vi "Stop.vi"(8 "error out":errorcluster, 10 "Wait (200ms)":u32=200, 11 "Generic Plugin in":refnum<class "Generic Plugin.lvclass">) -> (0 "error IO":errorcluster, 2 "Stopped Successfully (T) Aborted (F)":bool, 3 "Generic Plugin out":refnum<class "Generic Plugin.lvclass">)   [LabVIEW 2011, in "Generic Plugin.lvclass"]
uses:
  Plugin Template/Generic Plugin.lvclass
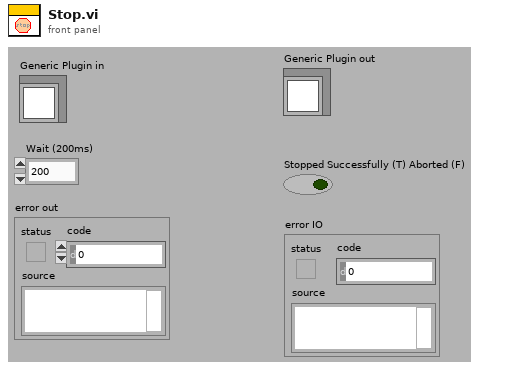
[diagram p1: front panel]
types:
  T1 = enum32{"Bad", "Idle", "Run top level", "Running"}
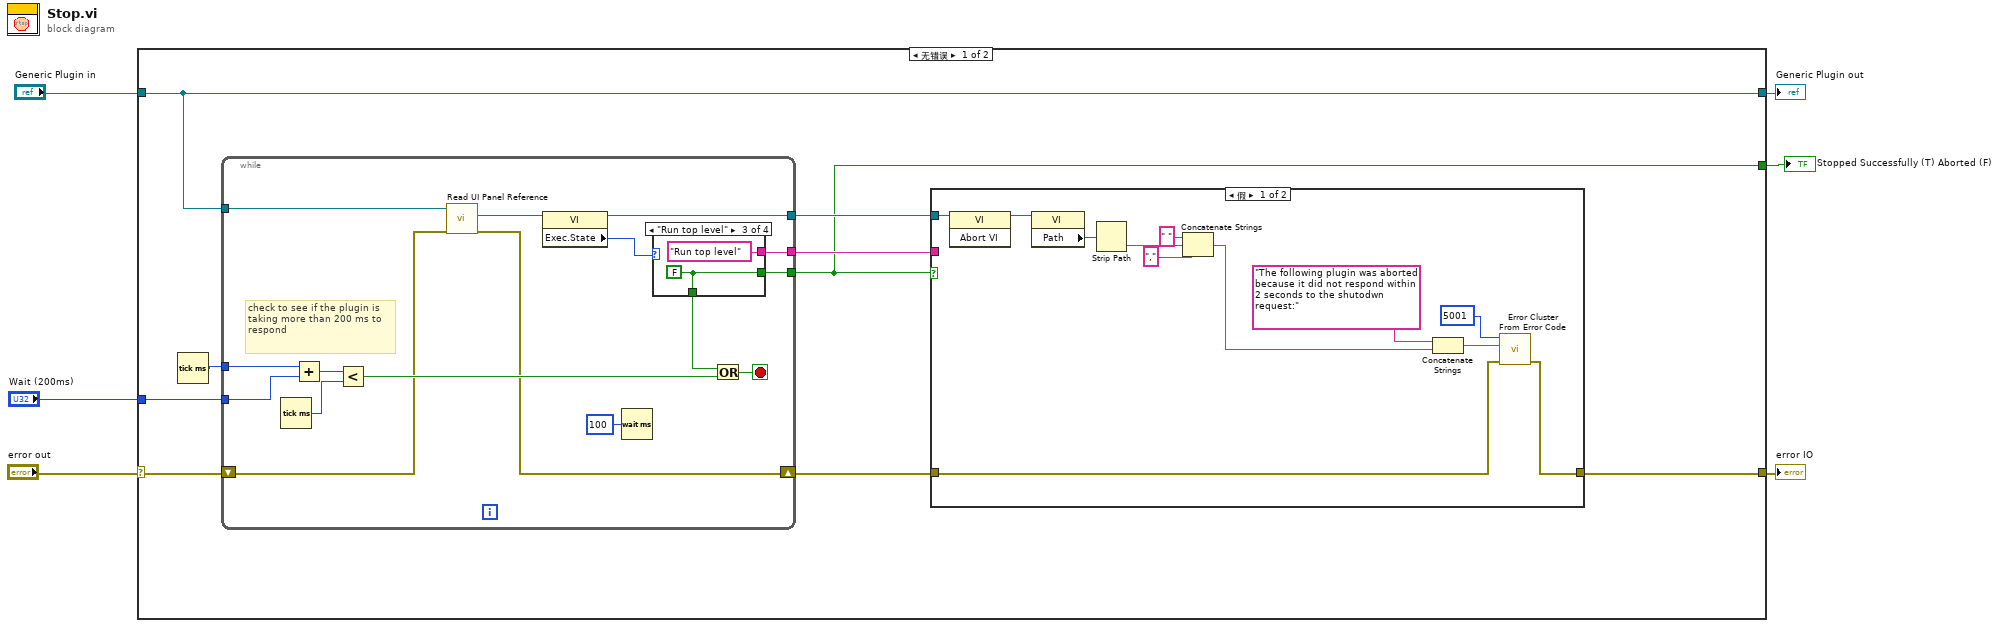
[diagram p0: block diagram]
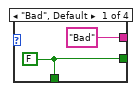
[diagram p3: hidden frame]
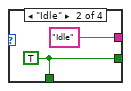
[diagram p4: hidden frame]
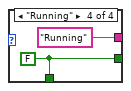
[diagram p5: hidden frame]
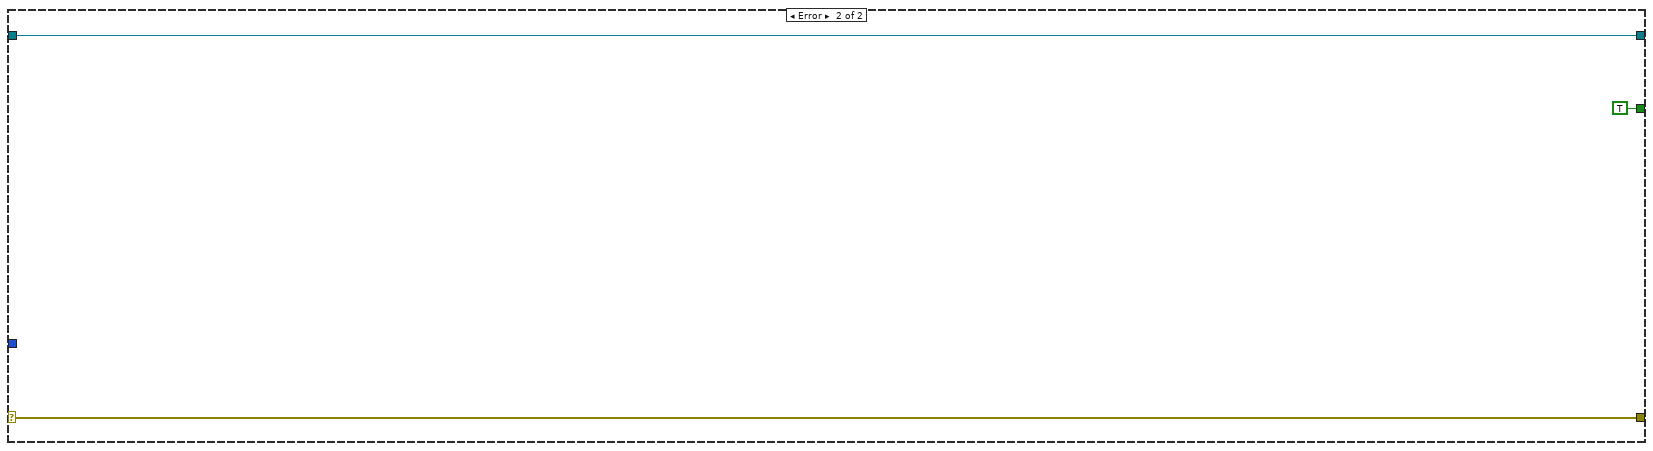
[diagram p6: hidden frame]
diagram:
  n1 = case shown="无错误" "error out" {
    selector: "error out" -> [w10 w55]
    tunnel: "Generic Plugin in" -> [w7 w53]
    tunnel: "Wait (200ms)" -> [w12 _]
    tunnel: [w9 w55] -> w3
    tunnel: [w8 TRUE ("x")] -> w2
    tunnel: [w7 w53] -> w1
    frame No Error {
      n2 = Tick Count (ms)() -> (millisecond timer value=w15:u32)
      n3 = while {
        tunnel: w7 -> [w44]
        tunnel: w15 -> [w43]
        tunnel: [w37] -> w8
        tunnel: [w35] -> w13
        tunnel: [w34] -> w14
        shift-right: [w31] -> w11
        shift-left: w10 -> [w32]
        tunnel: w12 -> [w30]
        stop <- w38 stop-if-true
        # "check to see if the plugin is\ntaking more than 200 ms to respond"
        n4 = Tick Count (ms)() -> (millisecond timer value=w41:u32)
        n5 = Add(x=w43, y=w30) -> (x+y=w42:u32)
        n6 = Less?(x=w42, y=w41) -> (x < y?=w40:bool)
        n7 = call "Read UI Panel Reference.vi"("error in (no error)"=w32, "Generic Plugin in"=w44) -> ("error out"=w31:errorcluster, "UI Panel Reference"=w33:refnum<vi>)  [unwired: 7 in, 1 out]
        n8 = property class="VI"(reference=w33) -> (reference out=w35:refnum<vi>, "Exec.State"=w39:T1)  [unwired: 1 in, 1 out]
        n9 = Wait (ms)(milliseconds to wait=u32 100) -> ()  [unwired: 1 out]
        n10 = case shown="\"Run top level\"" w39 {
          tunnel: [w46 w48 w50 w52] -> w37
          tunnel: [w46 w48 w50 w52] -> w36
          tunnel: ["Bad" ("string") "Idle" ("string") "Run top level" ("string") "Running" ("string")] -> w34
          frame "Bad", Default {
            w46 = FALSE ("x")
          }
          frame "Idle" {
            w48 = TRUE ("x")
          }
          frame "Run top level" {
            w50 = FALSE ("x")
          }
          frame "Running" {
            w52 = FALSE ("x")
          }
        }
        n11 = Or(x=w36, y=w40) -> (x .or. y?=w38:bool)
      }
      n12 = case shown="假" w8 {
        tunnel: w13 -> [w27 _]
        tunnel: w14 -> [_ _]
        tunnel: w11 -> [w17 w28]
        tunnel: [w16 w28] -> w9
        frame False {
          n13 = invoke class="VI" method="Abort VI"(reference=w27) -> (reference out=w26:refnum<vi>)  [unwired: 2 in, 2 out]
          n14 = property class="VI"(reference=w26) -> ("Path"=w25:path)  [unwired: 1 in, 2 out]
          n15 = Strip Path(path=w25) -> (name=w24:string)  [unwired: 1 out]
          n16 = Concatenate Strings(" " ("string"), w24, "," ("string")) -> (w18:string)
          n17 = Concatenate Strings("The following plugin was aborted because it did not respond within 2 seconds to the shutodwn request:" ("source"), w18) -> (w20:string)
          n18 = call <vilib>:"Error Cluster From Error Code.vi"("error in (no error)"=w17, "error message (\"\")"=w20, "error code (0)"=5001) -> ("error out"=w16:errorcluster)  [unwired: 6 in]
        }
        frame True {
        }
      }
    }
    frame Error {
    }
  }
  "error IO" <- w3
  "Stopped Successfully (T) Aborted (F)" <- w2
  "Generic Plugin out" <- w1
